vi "5_kb_plot_main.vi"() -> ()   [LabVIEW 2019]
uses:
  helper_vis/TypeDef_Velocity.ctl
  Shared VIs/TypeDef_TDMS_States.ctl
  <vilib>/myRIO/Common/Instrument Driver Framework/myRIO v1.0/Encoder/typedefs/Encoder Signal Mode.ctl
  Shared VIs/ModelSpecific/ETHMikeModel.ctl
  Shared VIs/ModelSpecific/ReadOnlyGlobalActions.ctl
  <vilib>/myRIO/Instrument Drivers/Onboard IO/AI/typedefs/AI Reference.ctl
  <vilib>/myRIO/Common/Instrument Driver Framework/Utilities/typedefs/myRIO Generic Hardware Reference.ctl
  <vilib>/myRIO/Common/Instrument Driver Framework/Utilities/typedefs/Hardware Version Enum.ctl
  <vilib>/myRIO/Common/Instrument Driver Framework/Utilities/typedefs/myRIO v1.0 Reference.ctl
  <vilib>/myRIO/Common/Instrument Driver Framework/Utilities/typedefs/Generic FPGA Reference.ctl
  <vilib>/myRIO/Common/Instrument Driver Framework/myRIO v1.0/AI/typedefs/AI Channels List.ctl
  <vilib>/myRIO/Common/Instrument Driver Framework/myRIO v1.0/AI/typedefs/AI Channels Enum.ctl
  <vilib>/myRIO/Common/Instrument Driver Framework/Utilities/typedefs/Analog Scaling Constants List.ctl
  <vilib>/myRIO/Common/Instrument Driver Framework/Utilities/typedefs/Analog Scaling Constants.ctl
  <vilib>/userDefined/High Color/nirio_resource_hc.ctl
  <vilib>/myRIO/Instrument Drivers/Onboard IO/AO/typedefs/AO Reference.ctl
  <vilib>/myRIO/Common/Instrument Driver Framework/myRIO v1.0/AO/typedefs/AO Channels List.ctl
  <vilib>/myRIO/Common/Instrument Driver Framework/myRIO v1.0/AO/typedefs/AO Channels Enum.ctl
  <vilib>/Platform/TimedLoop/XDataNode/timing_clust.ctl
  <vilib>/Platform/TimedLoop/XDataNode/nitl_modes.ctl
  <vilib>/Platform/TimedLoop/XDataNode/wakeup.ctl
  <vilib>/Analysis/3filter.llb/Filter Passband Type.ctl
  <vilib>/myRIO/Common/Instrument Driver Framework/myRIO v1.0/AI/vis/myRIO v1.1 Open AI.vi
  <vilib>/myRIO/Common/Instrument Driver Framework/myRIO v1.0/AO/vis/myRIO v1.1 Open AO.vi
  <vilib>/myRIO/Common/Instrument Driver Framework/Utilities/vis/Validate Channels.vi
  <vilib>/myRIO/Common/Instrument Driver Framework/myRIO v1.0/AI/vis/myRIO v1.0 Reserve AI.vi
  <vilib>/myRIO/Common/Instrument Driver Framework/myRIO v1.0/AO/vis/myRIO v1.0 Reserve AO.vi
  <vilib>/myRIO/Common/Instrument Driver Framework/myRIO v1.0/AI/vis/myRIO v1.0 Close AI.vi
  <vilib>/myRIO/Common/Instrument Driver Framework/myRIO v1.0/AO/vis/myRIO v1.0 Close AO.vi
  <vilib>/myRIO/Common/Instrument Driver Framework/myRIO v1.0/Encoder/vis/myRIO v1.0 Close Encoder.vi
  <vilib>/myRIO/Common/Instrument Driver Framework/myRIO v1.0/AI/vis/myRIO v1.0 Build MUX Configuration AI.vi
  <vilib>/myRIO/Common/Instrument Driver Framework/myRIO v1.0/Resource Manager/vis/myRIO v1.0 Reserve Channel List.vi
  <vilib>/myRIO/Common/Instrument Driver Framework/myRIO v1.0/AO/vis/myRIO v1.0 Build MUX Configuration AO.vi
  <vilib>/myRIO/Common/Instrument Driver Framework/myRIO v1.0/AI/vis/myRIO v1.0 Unreserve AI.vi
  <vilib>/myRIO/Common/Instrument Driver Framework/myRIO v1.0/AO/vis/myRIO v1.0 Unreserve AO.vi
  <vilib>/myRIO/Common/Instrument Driver Framework/myRIO v1.0/Encoder/vis/myRIO v1.0 Unreserve Encoder.vi
  <vilib>/myRIO/Common/Instrument Driver Framework/myRIO v1.0/Resource Manager/vis/myRIO v1.0 Reserve Channel.vi
  <vilib>/myRIO/Common/Instrument Driver Framework/myRIO v1.0/Resource Manager/vis/myRIO v1.0 Unreserve Channel.vi
  <vilib>/myRIO/Common/Instrument Driver Framework/myRIO v1.0/Resource Manager/vis/myRIO v1.0 Unreserve Channel List.vi
  <vilib>/myRIO/Common/Instrument Driver Framework/myRIO v1.0/Encoder/vis/myRIO v1.0 Build MUX Configuration Encoder.vi
  <vilib>/myRIO/Common/Instrument Driver Framework/myRIO v1.0/Resource Manager/vis/myRIO v1.0 Build Mutex Name.vi
  <vilib>/myRIO/Common/Instrument Driver Framework/myRIO v1.0/Resource Manager/vis/myRIO v1.0 Create Configuration List.vi
  <vilib>/Utility/VariantDataType/GetNumericInfo.vi
  <vilib>/Utility/error.llb/Error Cluster From Error Code.vi
  <vilib>/myRIO/Common/Instrument Driver Framework/myRIO v1.0/myRIO v1.1 Open.vi
  <vilib>/myRIO/Common/Instrument Driver Framework/myRIO v1.0/AO/vis/myRIO v1.0 Get Scaling Constants AO.vi
  <vilib>/myRIO/Common/Instrument Driver Framework/Utilities/vis/IO Manager.vi
  <vilib>/myRIO/Common/Instrument Driver Framework/Utilities/vis/Configuration Manager.vi
  <vilib>/myRIO/Common/Instrument Driver Framework/myRIO v1.0/myRIO v1.0 Close.vi
  <vilib>/myRIO/Common/Instrument Driver Framework/myRIO v1.0/AO/vis/myRIO v1.0 Write AO.vi
  <vilib>/myRIO/Common/Instrument Driver Framework/myRIO v1.0/AI/vis/myRIO v1.0 Get Scaling Constants AI.vi
  <vilib>/myRIO/Common/Instrument Driver Framework/myRIO v1.0/AI/vis/myRIO v1.0 Read AI.vi
  <vilib>/myRIO/Common/Instrument Driver Framework/myRIO v1.0/Encoder/vis/myRIO v1.0 Read Encoder.vi
  <vilib>/myRIO/Common/Instrument Driver Framework/myRIO v1.0/Encoder/vis/myRIO v1.0 Enable Encoder.vi
  <vilib>/myRIO/Common/Instrument Driver Framework/myRIO v1.0/Encoder/vis/myRIO v1.0 Shutdown Encoder.vi
  <vilib>/myRIO/Common/Instrument Driver Framework/myRIO v1.0/Resource Manager/vis/myRIO v1.0 Configure IO.vi
  <vilib>/myRIO/Instrument Drivers/Onboard IO/AO/vis/myRIO AO Open.xnode
  <vilib>/myRIO/Instrument Drivers/Onboard IO/AI/vis/myRIO AI Open.xnode
  <vilib>/platform/TimedLoop/XDataNode/XDataNode.xnode
  <vilib>/myRIO/Instrument Drivers/Onboard IO/Encoder/Encoder.lvlib
  <vilib>/myRIO/Instrument Drivers/Onboard IO/AO/AO.lvlib
  <vilib>/Platform/TimedLoop/XDataNode/XDNodeRunTimeDep.lvlib
  <vilib>/myRIO/Instrument Drivers/Onboard IO/AI/AI.lvlib
  <vilib>/Analysis/NI_AALBase.lvlib
  <vilib>/ptbypt/NI_PtbyPt.lvlib
panel:
  in  "Torque Constant [Nm/A]":dbl=137.0 format="%#_13g"
  in  "TDMS Storage File Input":string
  out "TDMS States":T1
  in  "stop":bool
  out "Time (s)":dbl
  in  "Save data?":bool
  out "Force unfiltered":dbl
  out "Force [N]":dbl
  out "Force chart [N]":dbl(graph)
  out "Iteration Duration":i64
  in  "Velocity Method":T2
  in  "start rendering":bool
  out "Current Setpoint [A]":dbl
  out "Velocity [deg/s]":dbl
  out "Velocity [deg/s] Chart":dbl(graph)
  out "Current [A]":dbl
  out "Current [A] Chart":dbl(graph)
  out "Position [deg]":dbl
  out "Position [deg] Chart":dbl(graph)
  in  "Wall Position (deg)":dbl
  in  "B":dbl
  in  "K":dbl
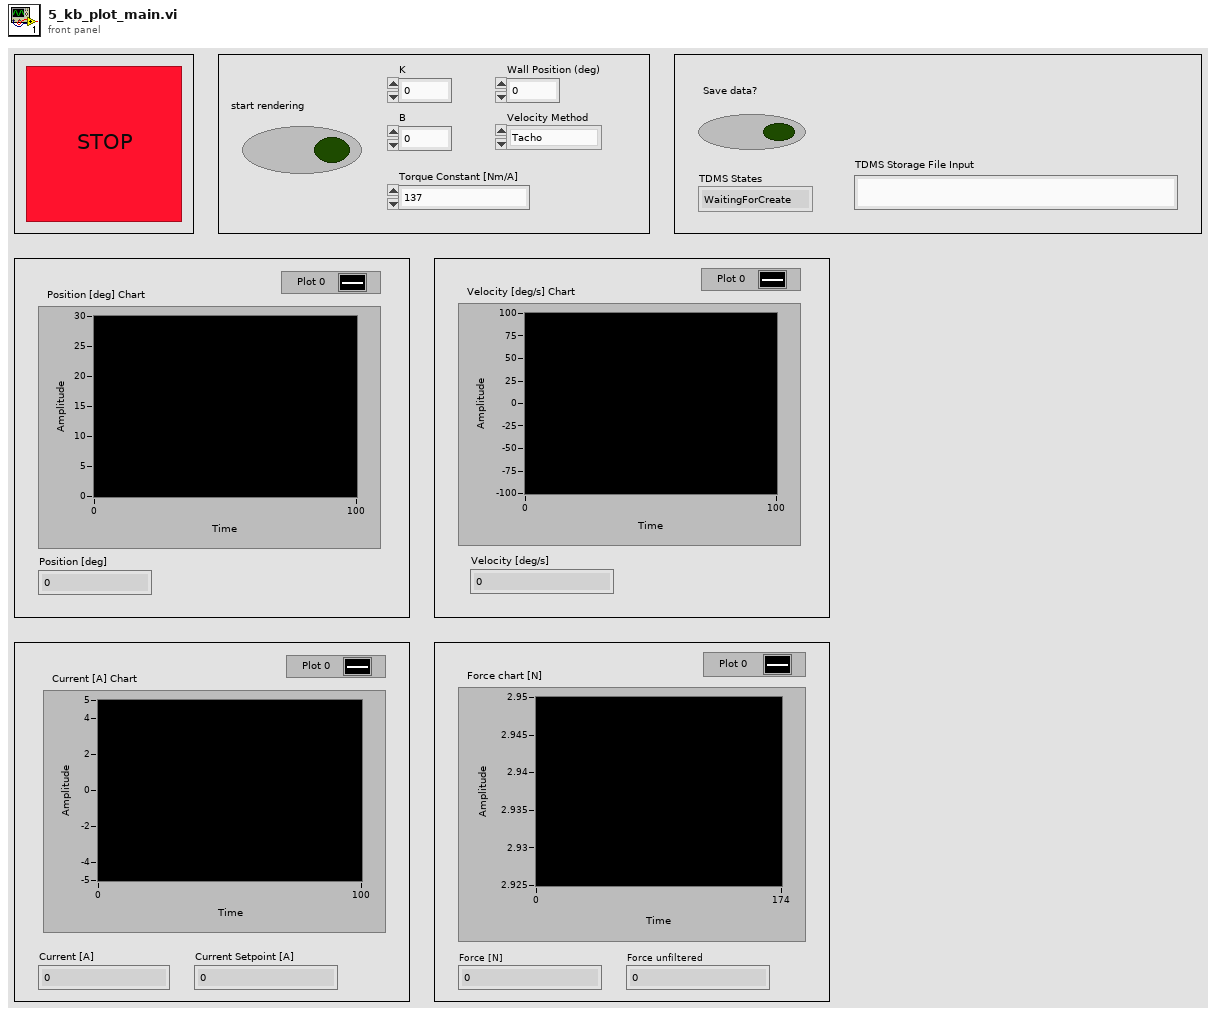
[diagram p1: front panel]
types:
  T1 = typedef "TypeDef_TDMS_States.ctl" = enum16{"WaitingForCreate", "Create", "Buffering", "Flushing", "Write", "Close"}
  T2 = typedef "TypeDef_Velocity.ctl" = enum16{"Tacho", "Encoder LP", "Encoder FOAW"}
  T3 = typedef "nirio_resource_hc.ctl" = tag
  T4 = typedef "Hardware Version Enum.ctl" = enum16{"Unknown", "myRIO-1900", "myRIO-1950", "roboRIO", "NI ELVIS RIO CM", "ELVIS III"}
  T5 = enum16{"open", "open or create", "create or replace", "create", "open (read-only)"}
  T6 = typedef "XDNodeRunTimeDep.lvlib/timing_clust.ctl" = cluster{"Expected End [f-1]":u64, "Actual End [f-1]":u64, "Finished Late? [f-1]":bool, "Expected End [i-1]":u64, "Actual End [i-1]":u64, "Finished Late? [i-1]":bool, "Expected Start [i]":u64, "Actual Start [i]":u64, "Expected Start [f]":u64, "Actual Start [f]":u64, "Source Name":string, "Structure Name":string, "Period":i64, "Deadline":i64, "Offset":i64, "Start":i64, "Priority":i32, "Timeout":i32, "Mode":T7, "Wakeup Reason":T8, "Error":errorcluster, "Source Type":string, "Secondary Source Type":string, "Global End Time":u64, "Global Start Time":u64, "Frame Duration":u64, "Iteration Duration":u64, "Assigned CPU":i32, "I/O Scan Engine Mode":u32}
  T7 = typedef "XDNodeRunTimeDep.lvlib/nitl_modes.ctl" = enum32{"No Change", "Process missed periods, maintain original phase", "Discard missed periods, maintain original phase", "Process missed periods, ignore original phase", "Discard missed periods, ignore original phase"}
  T8 = typedef "XDNodeRunTimeDep.lvlib/wakeup.ctl" = enum32{"Normal", "Aborted", "Asynchronous wakeup", "Timing source error", "Timed loop error", "Timeout"}
  T9 = typedef "NI_AALBase.lvlib/Filter Passband Type.ctl" = enum32{"Lowpass", "Highpass", "Bandpass", "Bandstop"}
  T10 = typedef "ReadOnlyGlobalActions.ctl" = enum16{"Initialize", "Read", "Write"}
  T11 = typedef "ETHMikeModel.ctl" = enum16{"ETH Mike #1", "ETH Mike #2", "ETH Mike #3", "ETH Mike #4", "ETH MIKE #5"}
  T12 = typedef "Encoder Signal Mode.ctl" = enum16{"Quadrature phase signal", "Step and direction signal"}
  T13 = typedef "AO.lvlib/AO Reference.ctl" = cluster{"myRIO Reference":T14, "AO Channel List":T17, "AO Scaling Constant List":T19}
  T14 = typedef "myRIO Generic Hardware Reference.ctl" = cluster{"myRIO Model":T4, "myRIO Hardware Reference":T15}
  T15 = typedef "myRIO v1.0 Reference.ctl" = cluster{"Generic FPGA Reference":T16, "Allow multiple opens":bool}
  T16 = typedef "Generic FPGA Reference.ctl" = refnum<k20>
  T17 = typedef "AO Channels List.ctl" = T18[]
  T18 = typedef "AO Channels Enum.ctl" = enum16{"Not Connected", "AudioOut/Left", "AudioOut/Right", "C/AO0", "C/AO1", "A/AO0", "A/AO1", "B/AO0", "B/AO1"}
  T19 = typedef "Analog Scaling Constants List.ctl" = T20[]
  T20 = typedef "Analog Scaling Constants.ctl" = cluster{"LSB Weight (Volts)":dbl, "Offset (Volts)":dbl, "Signed?":bool}
  T21 = typedef "AI.lvlib/AI Reference.ctl" = cluster{"myRIO Reference":T14, "AI Channels List":T22, "AI Scaling Constants List":T19}
  T22 = typedef "AI Channels List.ctl" = T23[]
  T23 = typedef "AI Channels Enum.ctl" = enum16{"Not Connected", "AudioIn/Left", "AudioIn/Right", "C/AI0", "C/AI1", "A/AI0", "A/AI1", "A/AI2", "A/AI3", "A/AI4", "A/AI5", "A/AI6", "A/AI7", "B/AI0", "B/AI1", "B/AI2", "B/AI3", "B/AI4", "B/AI5", "B/AI6", "B/AI7", "AI/AI0", "AI/AI1", "AI/AI2", "AI/AI3", "A/AI0 (DIFF)", "A/AI1 (DIFF)", "A/AI2 (DIFF)", "A/AI3 (DIFF)", "B/AI0 (DIFF)", "B/AI1 (DIFF)", "B/AI2 (DIFF)", "B/AI3 (DIFF)"}
  T24 = typedef "Encoder.lvlib/Encoder Reference.ctl" = cluster{"myRIO Reference":T14, "Encoder Channels Enum":T25}
  T25 = typedef "Encoder Channels Enum.ctl" = enum16{"Not Connected", "C/ENC0", "C/ENC1", "A/ENC", "A/ENC0", "A/ENC1", "A/ENC2", "A/ENC3", "A/ENC4", "A/ENC5", "A/ENC6", "A/ENC7", "A/ENC8", "A/ENC9", "B/ENC", "B/ENC0", "B/ENC1", "B/ENC2", "B/ENC3", "B/ENC4", "B/ENC5", "B/ENC6", "B/ENC7", "B/ENC8", "B/ENC9", "DIO/ENC0", "DIO/ENC1", "DIO/ENC2", "DIO/ENC3", "DIO/ENC4"}
  T26 = typedef "TypeDefTachometerParam.ctl" = cluster{"Offset [V]":dbl, "Gain [deg/sV]":dbl}
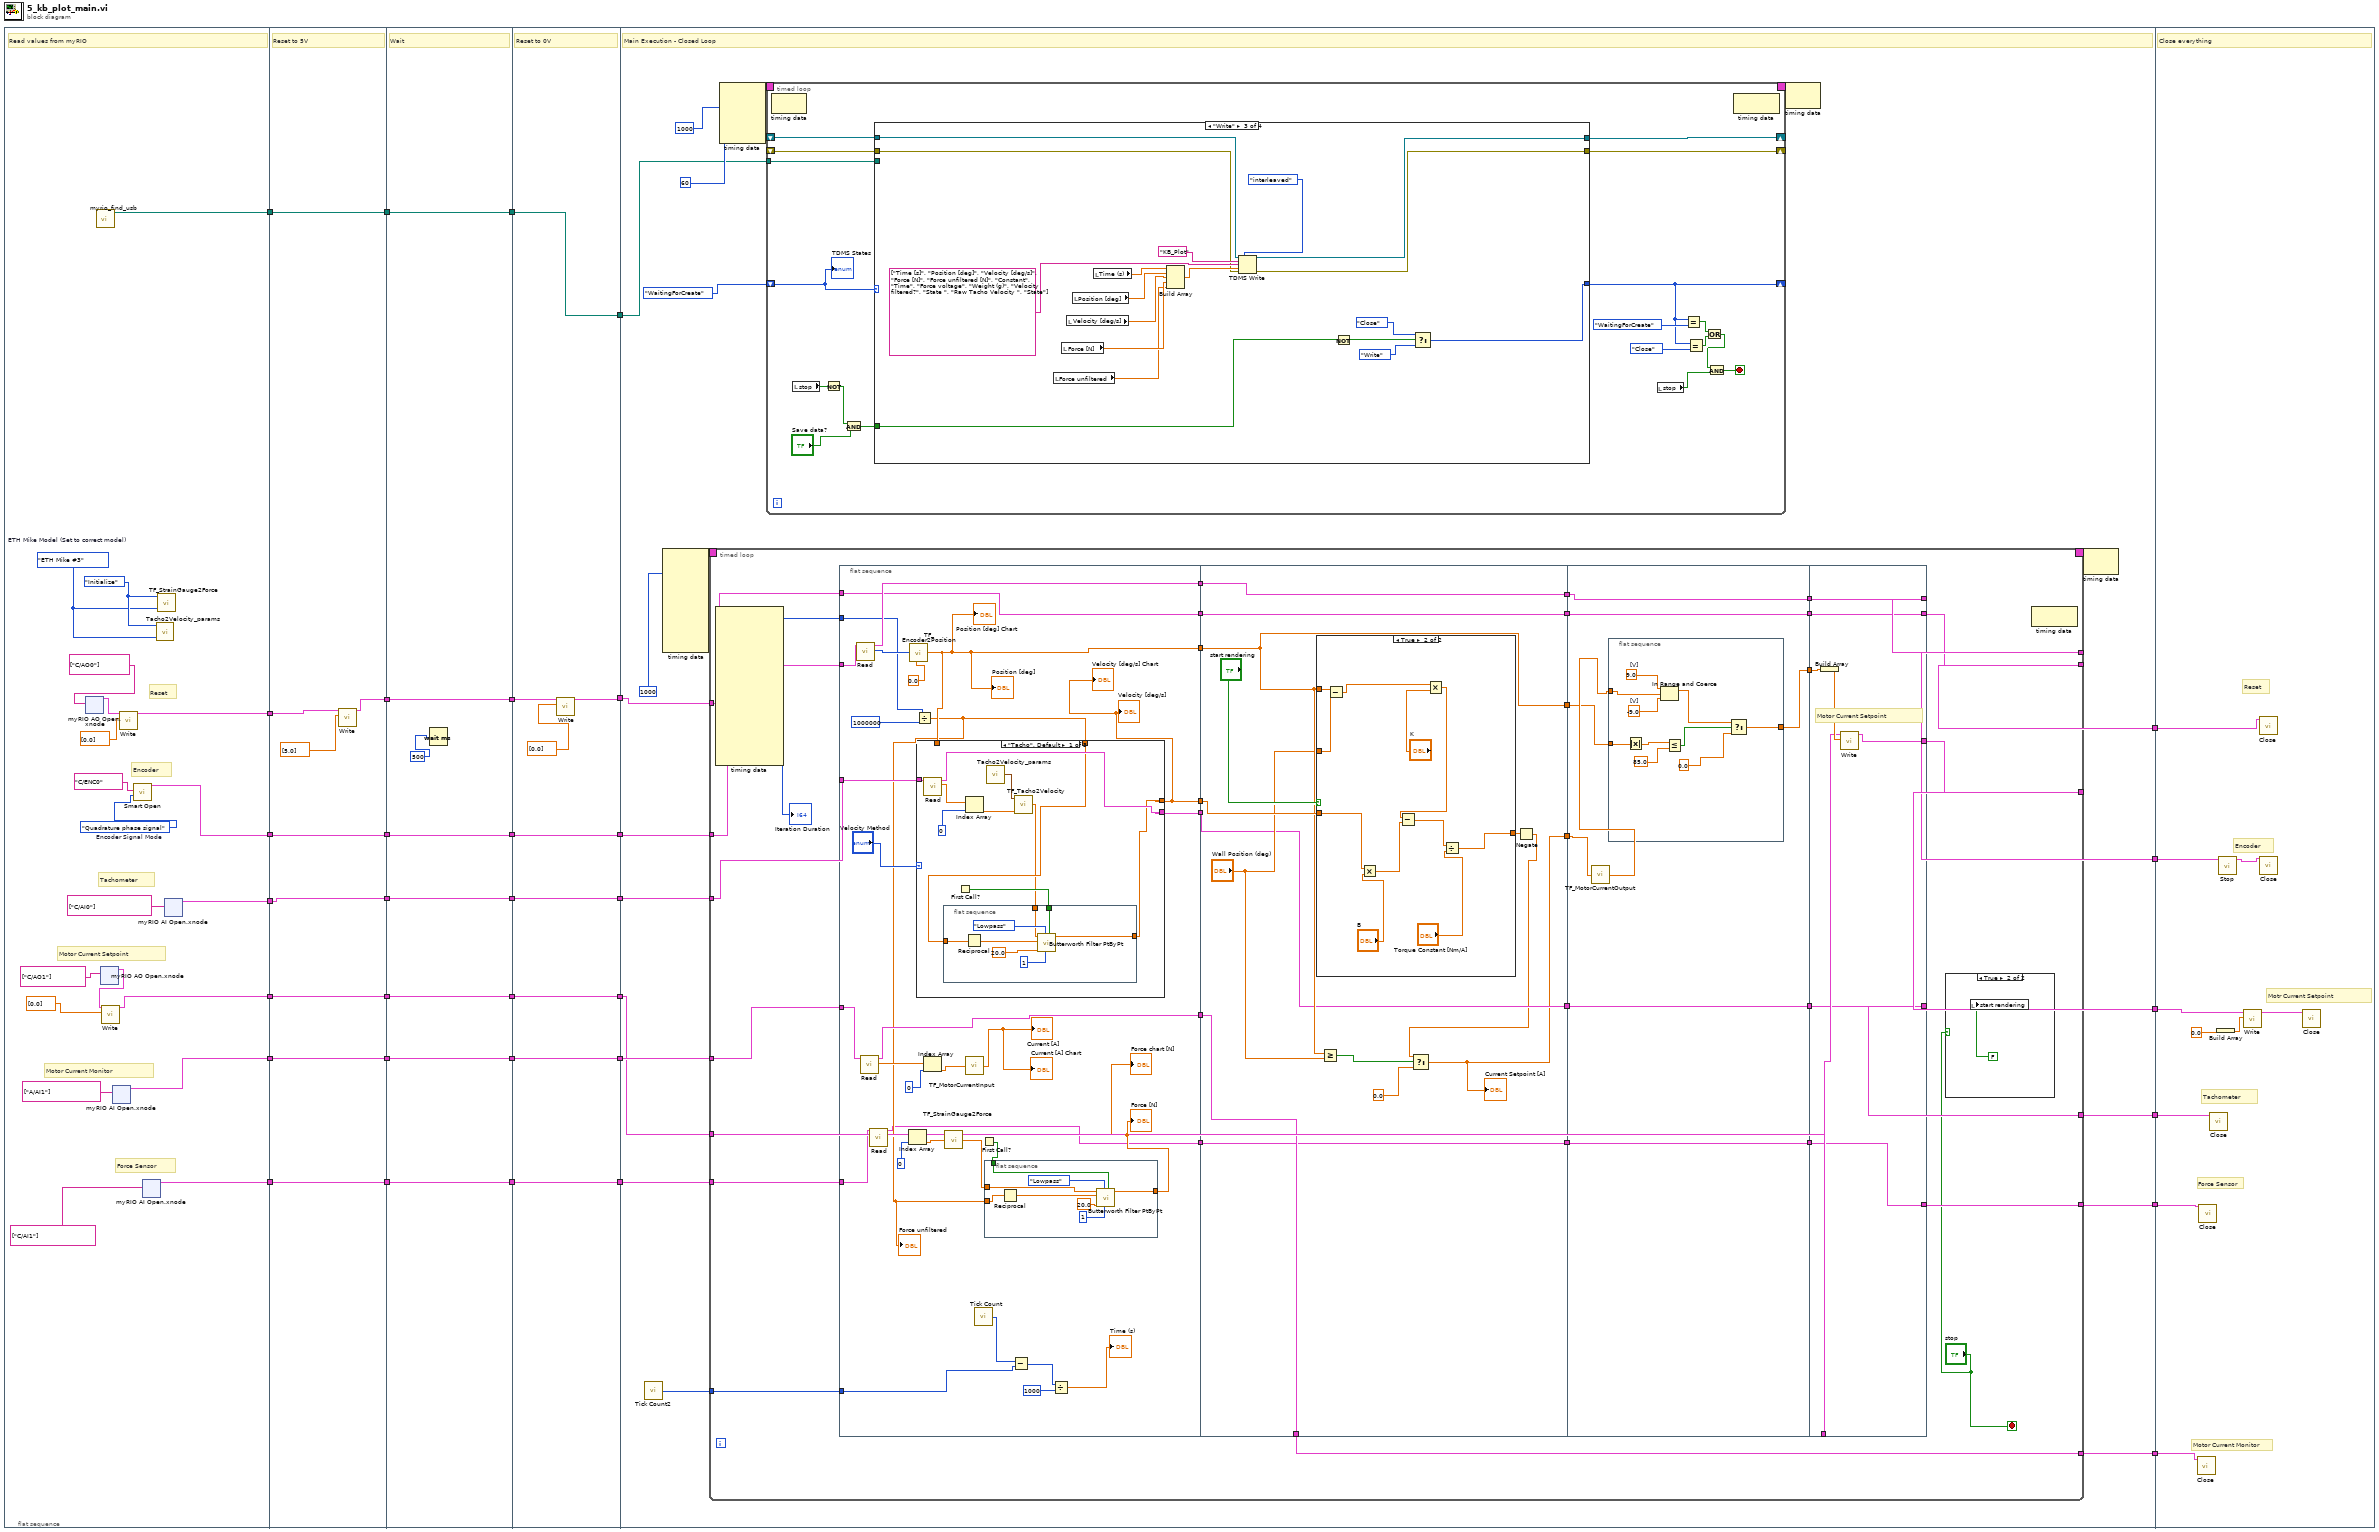
[diagram p0: block diagram]
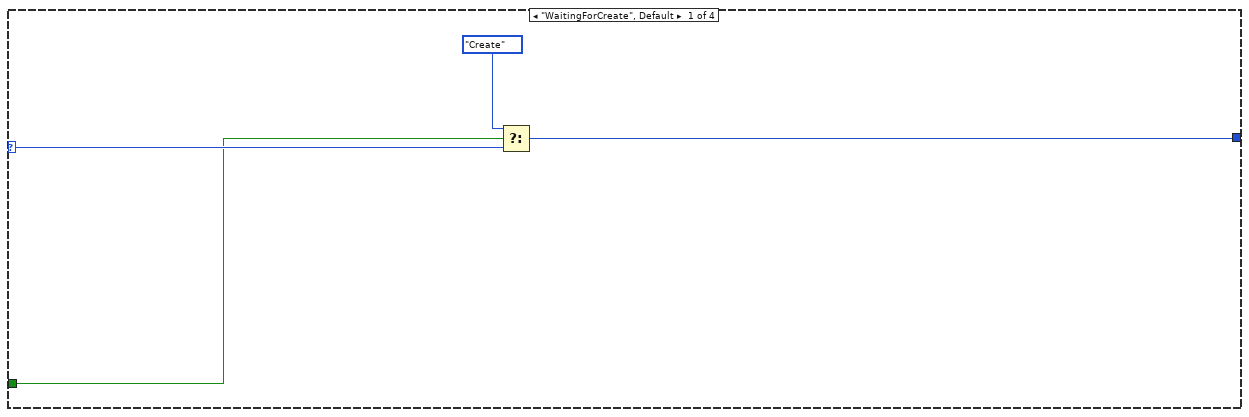
[diagram p2: hidden frame]
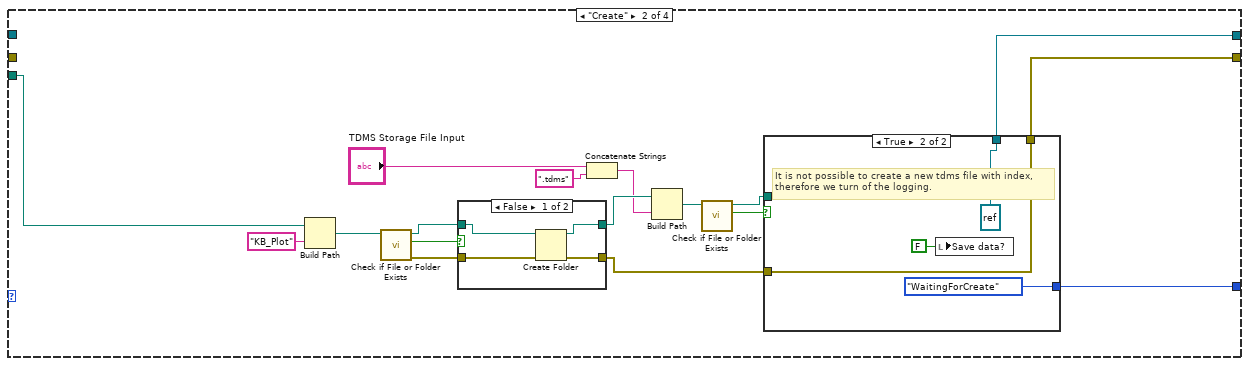
[diagram p3: hidden frame]
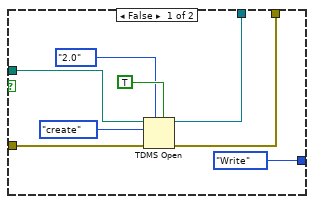
[diagram p4: hidden frame]
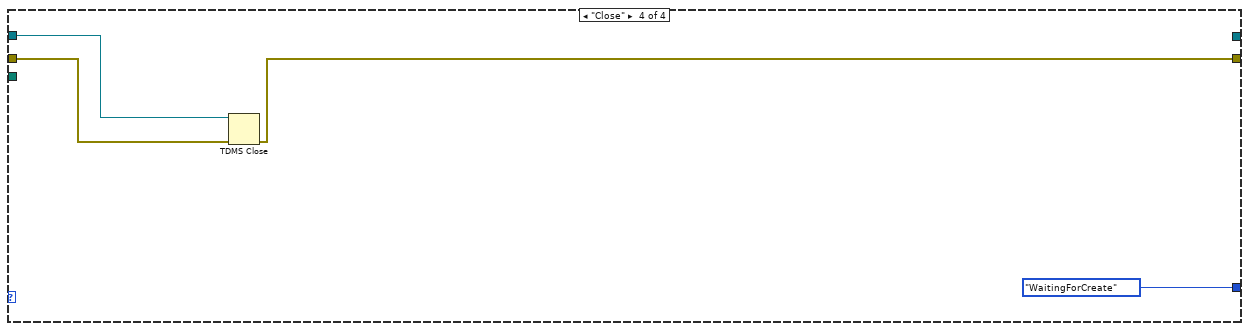
[diagram p6: hidden frame]
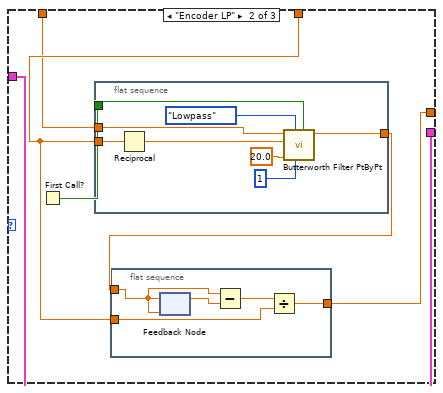
[diagram p8: hidden frame]
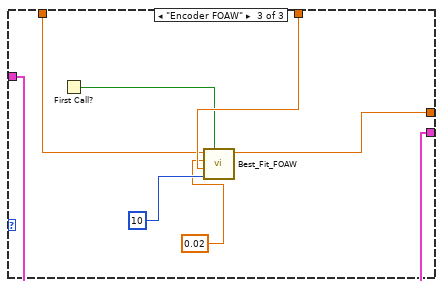
[diagram p9: hidden frame]
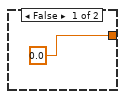
[diagram p10: hidden frame]
diagram:
  n1 = flat-sequence {
    tunnel: [w49] -> w34
    tunnel: [w48] -> w27
    tunnel: [w44] -> w26
    tunnel: [w42] -> w17
    tunnel: [w40] -> w16
    tunnel: [w38] -> w6
    tunnel: [w37] -> w2
    tunnel: w34 -> [w152]
    tunnel: [w151] -> w32
    tunnel: [w150] -> w28
    tunnel: w27 -> [w150]
    tunnel: w26 -> [w149]
    tunnel: [w149] -> w23
    tunnel: [w148] -> w18
    tunnel: w17 -> [w148]
    tunnel: w16 -> [w147]
    tunnel: [w147] -> w13
    tunnel: [w146] -> w7
    tunnel: w6 -> [w146]
    tunnel: [w145] -> w3
    tunnel: w2 -> [w145]
    tunnel: [w160] -> w33
    tunnel: w32 -> [w160]
    tunnel: [w159] -> w29
    tunnel: w28 -> [w159]
    tunnel: [w158] -> w24
    tunnel: w23 -> [w158]
    tunnel: [w157] -> w19
    tunnel: w18 -> [w157]
    tunnel: [w156] -> w14
    tunnel: w13 -> [w156]
    tunnel: [w155] -> w8
    tunnel: w7 -> [w155]
    tunnel: [w154] -> w4
    tunnel: w3 -> [w154]
    tunnel: w33 -> [w169]
    tunnel: [w168] -> w31
    tunnel: [w167] -> w30
    tunnel: w29 -> [w167]
    tunnel: [w166] -> w25
    tunnel: w24 -> [w166]
    tunnel: [w165] -> w20
    tunnel: w19 -> [w165]
    tunnel: [w164] -> w15
    tunnel: w14 -> [w164]
    tunnel: [w163] -> w9
    tunnel: w8 -> [w163]
    tunnel: [w162] -> w5
    tunnel: w4 -> [w162]
    tunnel: w31 -> [w183]
    tunnel: w30 -> [w189]
    tunnel: w25 -> [w185]
    tunnel: [w182] -> w22
    tunnel: [w184] -> w21
    tunnel: w20 -> [w188]
    tunnel: w15 -> [w187]
    tunnel: [w186] -> w12
    tunnel: [w181] -> w11
    tunnel: [w180] -> w10
    tunnel: w9 -> [w179]
    tunnel: w5 -> [w174]
    tunnel: [w173] -> w1
    tunnel: w22 -> [w463]
    tunnel: w21 -> [w462]
    tunnel: w12 -> [w461]
    tunnel: w11 -> [w460]
    tunnel: w10 -> [w459]
    tunnel: w1 -> [w458]
    frame #0 {
      w36 = ReadOnlyGlobalActions."Initialize" ("Action (Read)")
      w35 = ETHMikeModel."ETH Mike #3"  # ETH Mike Model (Set to correct model)
      w53 = Encoder_Signal_Mode."Quadrature phase signal"  # Encoder Signal Mode
      # "Force Sensor"
      # "Tachometer"
      # "Motor Current Monitor"
      # "Motor Current Setpoint"
      # "Reset"
      # "Encoder"
      # "Read values from myRIO"
      n2 = xnode "myRIO AO Open.xnode"("Channel Names"=tag[] ["C/AO0"]) -> ("AO Ref Out"=w51:T13)  [unwired: 2 in, 1 out]
      n3 = call "myrio_find_usb.vi"() -> ("Largest USB Partition Path"=w37:path)  [unwired: 9 in, 2 out]
      n4 = xnode "myRIO AO Open.xnode"("Channel Names"=tag[] ["C/AO1"]) -> ("AO Ref Out"=w46:T13)  [unwired: 2 in, 1 out]
      n5 = call <vilib>:"Write.vi"("Values"=dbl[] [0.0], "AO Ref In"=w46) -> ("AO Ref Out"=w44:T13)  [unwired: 7 in, 1 out]
      n6 = xnode "myRIO AI Open.xnode"("Channel Names"=tag[] ["A/AI1"]) -> ("AI Ref Out"=w42:T21)  [unwired: 2 in, 1 out]
      n7 = call <vilib>:"Write.vi"("Values"=dbl[] [0.0], "AO Ref In"=w51) -> ("AO Ref Out"=w49:T13)  [unwired: 7 in, 1 out]
      n8 = call <vilib>:"Smart Open.vi"("Encoder Signal Mode"=w53, "Channel Name"=tag "C/ENC0") -> ("Encoder Ref Out"=w48:T24)  [unwired: 8 in, 1 out]
      n9 = xnode "myRIO AI Open.xnode"("Channel Names"=tag[] ["C/AI1"]) -> ("AI Ref Out"=w38:T21)  [unwired: 2 in, 1 out]
      n10 = call "Tacho2Velocity_params.vi"("Action (Read)"=w36, "ETH Mike Model"=w35) -> ()  [unwired: 3 in, 1 out]
      n11 = call "TF_StrainGauge2Force.vi"("Action (Read)"=w36, "ETH Mike Model"=w35) -> ()  [unwired: 3 in, 1 out]
      n12 = xnode "myRIO AI Open.xnode"("Channel Names"=tag[] ["C/AI0"]) -> ("AI Ref Out"=w40:T21)  [unwired: 2 in, 1 out]
    }
    frame #1 {
      # "Reset to 5V"
      n13 = call <vilib>:"Write.vi"("Values"=dbl[] [5.0], "AO Ref In"=w152) -> ("AO Ref Out"=w151:T13)  [unwired: 7 in, 1 out]
    }
    frame #2 {
      # "Wait"
      n14 = Wait (ms)(milliseconds to wait=500) -> ()  [unwired: 1 out]
    }
    frame #3 {
      # "Reset to 0V"
      n15 = call <vilib>:"Write.vi"("Values"=dbl[] [0.0], "AO Ref In"=w169) -> ("AO Ref Out"=w168:T13)  [unwired: 7 in, 1 out]
    }
    frame #4 {
      # "Main Execution - Closed Loop"
      n16 = call "Tick Count2"() -> ("Tick Count(mSec)"=w172:u32)
      n17 = node-c288(1000) -> (w192:T6)  [unwired: 9 in]
      n18 = timed-loop {
        timing: w192 -> [_]
        timing-out: [_] -> w191
        tunnel: w189 -> [w305]
        tunnel: w188 -> [w312]
        tunnel: w187 -> [w311]
        tunnel: [w306] -> w186
        tunnel: w185 -> [w304]
        tunnel: [w300] -> w184
        tunnel: w183 -> [w299]
        tunnel: [w295] -> w182
        tunnel: [w291] -> w181
        tunnel: [w289] -> w180
        tunnel: w179 -> [w286]
        tunnel: [w284] -> w173
        tunnel: w172 -> [w280]
        stop <- "stop" stop-if-true
        n19 = node-c288() -> (w290:i64, →"Iteration Duration":i64)  [unwired: 1 in, 15 out]
        n20 = flat-sequence {
          tunnel: w305 -> [w345]
          tunnel: w312 -> [w342]
          tunnel: w311 -> [w337]
          tunnel: [w330] -> w310
          tunnel: [w329] -> w309
          tunnel: [w336] -> w302
          tunnel: w299 -> [w335]
          tunnel: [w335] -> w296
          tunnel: [w334] -> w294
          tunnel: w290 -> [w333]
          tunnel: [w328] -> w288
          tunnel: w286 -> [w327]
          tunnel: [w319] -> w281
          tunnel: w280 -> [w317]
          tunnel: w310 -> [w407]
          tunnel: w309 -> [w411]
          tunnel: [w399] -> w308
          tunnel: [w407] -> w307
          tunnel: [w410] -> w303
          tunnel: w302 -> [w410]
          tunnel: [w409] -> w297
          tunnel: w296 -> [w409]
          tunnel: w294 -> [w401]
          tunnel: [w401] -> w292
          tunnel: [w402] -> w289
          tunnel: w288 -> [w402]
          tunnel: [w398] -> w282
          tunnel: w281 -> [w398]
          tunnel: w308 -> [w431]
          tunnel: w307 -> [w426]
          tunnel: w303 -> [w430]
          tunnel: [w430] -> w301
          tunnel: [w429] -> w298
          tunnel: w297 -> [w429]
          tunnel: [w428] -> w293
          tunnel: w292 -> [w428]
          tunnel: [w425] -> w285
          tunnel: [w424] -> w283
          tunnel: w282 -> [w424]
          tunnel: [w448] -> w306
          tunnel: w304 -> [w447]
          tunnel: [w446] -> w300
          tunnel: w301 -> [w446]
          tunnel: w298 -> [w445]
          tunnel: [w445] -> w295
          tunnel: [w444] -> w291
          tunnel: w293 -> [w444]
          tunnel: w285 -> [w443]
          tunnel: [w442] -> w284
          tunnel: w283 -> [w442]
          frame #0 {
            n21 = call <vilib>:"Read.vi"("Encoder Ref In"=w345) -> ("Counter Value"=w344:i32, "Encoder Ref Out"=w336:T24)  [unwired: 6 in, 3 out]
            n22 = call <vilib>:"Read.vi"("AI Ref In"=w342) -> ("Values"=w341:dbl[], "AI Ref Out"=w328:T21)  [unwired: 8 in, 1 out]
            n23 = call <vilib>:"Read.vi"("AI Ref In"=w327) -> ("Values"=w326:dbl[], "AI Ref Out"=w319:T21)  [unwired: 8 in, 1 out]
            n24 = Index Array(array=w326, index=0) -> (element=w324:dbl)
            n25 = call "TF_Encoder2Position.vi"("Counter Value"=w344, "Offset"=0.0) -> ("Position [deg]"=w330:dbl)  [unwired: 3 in]
            "Position [deg] Chart" <- w330
            "Position [deg]" <- w330
            n26 = Divide(x=w333, y=1000000) -> (x/y=w320:dbl)
            "Force unfiltered" <- w320
            n27 = case shown="\"Tacho\", Default" "Velocity Method" {
              tunnel: w337 -> [w363 w377 w391]
              tunnel: [w360 w377 w391] -> w334
              tunnel: w320 -> [w359 w375 w396]
              tunnel: [w357 w374 w392] -> w329
              tunnel: w330 -> [_ w373 w394]
              frame "Tacho", Default {
                n28 = call <vilib>:"Read.vi"("AI Ref In"=w363) -> ("Values"=w361:dbl[], "AI Ref Out"=w360:T21)  [unwired: 8 in, 1 out]
                n29 = flat-sequence {
                  tunnel: w359 -> [w370]
                  tunnel: [w366] -> w357
                  tunnel: w358 -> [w365]
                  tunnel: w354 -> [w364]
                  frame #0 {
                    n30 = Reciprocal(x=w370) -> (1/x=w371:dbl)
                    n31 = call <vilib>:"Butterworth Filter PtByPt.vi"("initialize"=w365, "order"=1, "filter type"=Filter_Passband_Type."Lowpass", "low cutoff freq: fl"=20.0, "sampling freq: fs"=w371, "x"=w364) -> ("Filtered x"=w366:dbl)  [unwired: 3 in, 1 out]
                  }
                }
                n32 = First Call?() -> (First Call?: T/F=w358:bool)
                n33 = Index Array(array=w361, index=0) -> (element=w355:dbl)
                n34 = call "Tacho2Velocity_params.vi"() -> ("Cluster"=w356:T26)  [unwired: 5 in]
                n35 = call "TF_Tacho2Velocity.vi"("Tachometer Voltage [V]"=w355, "Tachometer param"=w356) -> ("Tachometer Velocity [deg/s]"=w354:dbl)  [unwired: 2 in]
              }
              frame "Encoder LP" {
                n36 = First Call?() -> (First Call?: T/F=w376:bool)
                n37 = flat-sequence {
                  tunnel: w373 -> [w390]
                  tunnel: w375 -> [w388]
                  tunnel: w376 -> [w385]
                  tunnel: [w383] -> w372
                  frame #0 {
                    n38 = Reciprocal(x=w388) -> (1/x=w389:dbl)
                    n39 = call <vilib>:"Butterworth Filter PtByPt.vi"("initialize"=w385, "order"=1, "filter type"=Filter_Passband_Type."Lowpass", "low cutoff freq: fl"=20.0, "sampling freq: fs"=w389, "x"=w390) -> ("Filtered x"=w383:dbl)  [unwired: 3 in, 1 out]
                  }
                }
                n40 = flat-sequence {
                  tunnel: w375 -> [w380]
                  tunnel: [w379] -> w374
                  tunnel: w372 -> [w378]
                  frame #0 {
                    n41 = feedback #1(w378) -> (w382:dbl)
                    n42 = feedback-in #1(w378) -> ()
                    n43 = Subtract(x=w378, y=w382) -> (x-y=w381:dbl)
                    n44 = Divide(x=w381, y=w380) -> (x/y=w379:dbl)
                  }
                }
              }
              frame "Encoder FOAW" {
                n45 = First Call?() -> (First Call?: T/F=w393:bool)
                n46 = call "Best_Fit_FOAW.vi"("y_k"=w394, "d"=0.02, "T"=w396, "n_max"=10, "Initialize"=w393) -> ("vel estimation"=w392:dbl)  [unwired: 4 in, 1 out]
              }
            }
            "Velocity [deg/s]" <- w329
            "Velocity [deg/s] Chart" <- w329
            n47 = Index Array(array=w341, index=0) -> (element=w339:dbl)
            n48 = call "TF_StrainGauge2Force.vi"("Strain Gauge Value [V]"=w324) -> ("Force [N]"=w323:dbl)  [unwired: 4 in]
            n49 = call "TF_MotorCurrentInput.vi"("Motor Current Monitor Value [V]"=w339) -> ("Current [A]"=→"Current [A] Chart" →"Current [A]":dbl)
            n50 = call "Tick Count"() -> ("Tick Count(mSec)"=w318:u32)
            n51 = First Call?() -> (First Call?: T/F=w322:bool)
            n52 = flat-sequence {
              tunnel: w323 -> [w353]
              tunnel: [w348] -> w321
              tunnel: w320 -> [w347]
              tunnel: w322 -> [w346]
              frame #0 {
                n53 = Reciprocal(x=w347) -> (1/x=w352:dbl)
                n54 = call <vilib>:"Butterworth Filter PtByPt.vi"("initialize"=w346, "order"=1, "filter type"=Filter_Passband_Type."Lowpass", "low cutoff freq: fl"=20.0, "sampling freq: fs"=w352, "x"=w353) -> ("Filtered x"=w348:dbl)  [unwired: 3 in, 1 out]
              }
            }
            n55 = Subtract(x=w318, y=w317) -> (x-y=w316:u32)
            n56 = Divide(x=w316, y=u32 1000) -> (x/y=→"Time (s)":dbl)
            "Force [N]" <- w321
            "Force chart [N]" <- w321
          }
          frame #1 {
            n57 = case shown="True" "start rendering" {
              tunnel: w411 -> [_ w420]
              tunnel: [0.0 w415] -> w403
              tunnel: w407 -> [_ w414]
              tunnel: "Wall Position (deg)" -> [_ w413]
              frame False {
              }
              frame True {
                n58 = Subtract(x=w414, y=w413) -> (x-y=w422:dbl)
                n59 = Multiply(x=w420, y="B") -> (x*y=w418:dbl)
                n60 = Multiply(x=w422, y="K") -> (x*y=w421:dbl)
                n61 = Subtract(x=w421, y=w418) -> (x-y=w416:dbl)
                n62 = Divide(x=w416, y="Torque Constant [Nm/A]") -> (x/y=w415:dbl)
              }
            }
            n63 = Greater Or Equal?(x=w407, y="Wall Position (deg)") -> (x >= y?=w406:bool)
            n64 = Negate(x=w403) -> (-x=w400:dbl)
            n65 = Select(t=w400, s=w406, f=0.0) -> (s? t:f=w399:dbl)
            "Current Setpoint [A]" <- w399
          }
          frame #2 {
            n66 = call "TF_MotorCurrentOutput.vi"("Motor Current Setpoint [A]"=w431) -> ("Motor Current Setpoint [V]"=w427:dbl)
            n67 = flat-sequence {
              tunnel: w426 -> [w437]
              tunnel: w427 -> [w433]
              tunnel: [w432] -> w425
              frame #0 {
                w441 = -9.0  # [V]
                w440 = 9.0  # [V]
                n68 = Absolute Value(x=w437) -> (abs(x)=w438:dbl)
                n69 = In Range and Coerce(upper limit=w440, x=w433, lower limit=w441) -> (coerced(x)=w439:dbl)  [unwired: 1 out]
                n70 = Less Or Equal?(x=w438, y=85.0) -> (x <= y?=w435:bool)
                n71 = Select(t=w439, s=w435, f=0.0) -> (s? t:f=w432:dbl)
              }
            }
          }
          frame #3 {
            # "Motor Current Setpoint"
            n72 = Build Array(w443) -> (w449:dbl[])
            n73 = call <vilib>:"Write.vi"("Values"=w449, "AO Ref In"=w447) -> ("AO Ref Out"=w448:T13)  [unwired: 7 in, 1 out]
          }
        }
        n74 = case shown="True" "stop" {
          frame False {
          }
          frame True {
            n75 = local write "start rendering"(FALSE ("start measurement")) -> ()
          }
        }
        n76 = node-c288() -> ()  [unwired: 1 in, 1 out]
      }
      n77 = node-c288(i64 1000 ("Period"), 60) -> (w178:T6)  [unwired: 3 in]
      n78 = timed-loop {
        timing: w178 -> [_]
        timing-out: [_] -> w177
        tunnel: w174 -> [w210]
        shift-right: [w209] -> _
        shift-left: _ -> [w208]
        shift-right: [w207] -> _
        shift-left: _ -> [w206]
        shift-right: [w196] -> _
        shift-left: TypeDef_TDMS_States."WaitingForCreate" ("TDMS States") -> [w201]
        stop <- w193 stop-if-true
        n79 = node-c288() -> ()  [unwired: 1 in, 1 out]
        n80 = local read "stop"() -> (w205:bool)
        n81 = Not(x=w205) -> (.not. x?=w203:bool)
        n82 = And(x=w203, y="Save data?") -> (x .and. y?=w202:bool)
        n83 = case shown="\"Write\"" w201 {
          selector: w201 -> [w214 _ _ _]
          tunnel: w202 -> [w213 _ w251 _]
          tunnel: w210 -> [_ w222 _ _]
          tunnel: [_ w217 w256 w269] -> w209
          tunnel: w208 -> [_ _ w259 w270]
          tunnel: [_ w216 w255 _] -> w207
          tunnel: w206 -> [_ _ w258 w271]
          tunnel: [w211 w219 w250 TypeDef_TDMS_States."WaitingForCreate" ("TDMS States")] -> w196
          frame "WaitingForCreate", Default {
            n84 = Select(t=TypeDef_TDMS_States."Create" ("TDMS States"), s=w213, f=w214) -> (s? t:f=w211:T1)
          }
          frame "Create" {
            n85 = Build Path(base path=w222, name or relative path="KB_Plot") -> (appended path=w224:path)
            n86 = call <vilib>:"Check if File or Folder Exists.vi"("path"=w224) -> ("error out"=w229:errorcluster, "file or folder exists?"=w231:bool, "dup path"=w230:path)  [unwired: 8 in]
            n87 = case shown="False" w231 {
              tunnel: w230 -> [w247 w248]
              tunnel: [w246 w249] -> w218
              tunnel: w229 -> [w245 w249]
              tunnel: [w244 w248] -> w228
              frame False {
                n88 = Create Folder(path (use dialog)=w247, error in=w245) -> (created path=w244:path, error out=w246:errorcluster)  [unwired: 1 in, 1 out]
              }
              frame True {
              }
            }
            n89 = Concatenate Strings("TDMS Storage File Input", ".tdms") -> (w225:string)
            n90 = Build Path(base path=w228, name or relative path=w225) -> (appended path=w221:path)
            n91 = call <vilib>:"Check if File or Folder Exists.vi"("path"=w221) -> ("file or folder exists?"=w220:bool, "dup path"=w215:path)  [unwired: 8 in, 1 out]
            n92 = case shown="True" w220 {
              tunnel: [TypeDef_TDMS_States."Write" ("TDMS States") TypeDef_TDMS_States."WaitingForCreate" ("TDMS States")] -> w219
              tunnel: w218 -> [w235 w240]
              tunnel: [w234 w240] -> w217
              tunnel: [w233 refnum<k34> refnum ("tdms file out")] -> w216
              tunnel: w215 -> [w232 _]
              frame False {
                n93 = TDMS Open(5:TRUE, 7:enum16{"1.0", "2.0"}."2.0" ("file format version (2.0)"), 8:w235, 10:T5."create" ("operation (0:open)"), 11:w232) -> (0:w234:errorcluster, 3:w233:refnum<k34>)  [unwired: 2 in]
              }
              frame True {
                # "It is not possible to create a new tdms file with index,\ntherefore we turn of the logging."
                n94 = local write "Save data?"(FALSE ("Save data?")) -> ()
              }
            }
          }
          frame "Write" {
            n95 = local read "Force unfiltered"() -> (w263:dbl)
            n96 = local read "Force [N]"() -> (w264:dbl)
            n97 = local read "Velocity [deg/s]"() -> (w265:dbl)
            n98 = local read "Position [deg]"() -> (w266:dbl)
            n99 = local read "Time (s)"() -> (w267:dbl)
            n100 = Build Array(w267, w266, w265, w264, w263) -> (w262:dbl[])
            n101 = TDMS Write(0:w258, 1:enum16{"decimated", "interleaved"}."interleaved" ("data layout (0:decimated)"), 5:"KB_Plot" ("group name in (Untitled)"), 7:string[] ["Time [s]", "Position [deg]", "Velocity [deg/s]", "Force [N]", "Force unfiltered [N]", "Constant", "Time", "Force voltage", "Weight (g)", "Velocity filtered?", "State ", "Raw Tacho Velocity ", "State"], 9:w262, 11:w259) -> (4:w255:refnum<k34>, 15:w256:errorcluster)  [unwired: 2 out]
            n102 = Not(x=w251) -> (.not. x?=w254:bool)
            n103 = Select(t=TypeDef_TDMS_States."Close" ("TDMS States"), s=w254, f=TypeDef_TDMS_States."Write" ("TDMS States")) -> (s? t:f=w250:T1)
          }
          frame "Close" {
            n104 = TDMS Close(8:w270, 11:w271) -> (0:w269:errorcluster)  [unwired: 1 out]
          }
        }
        n105 = local read "stop"() -> (w194:bool)
        n106 = Equal?(x=w196, y=TypeDef_TDMS_States."WaitingForCreate" ("TDMS States")) -> (x = y?=w198:bool)
        n107 = Equal?(x=w196, y=TypeDef_TDMS_States."Close" ("TDMS States")) -> (x = y?=w197:bool)
        n108 = Or(x=w198, y=w197) -> (x .or. y?=w195:bool)
        n109 = And(x=w195, y=w194) -> (x .and. y?=w193:bool)
        n110 = node-c288() -> ()  [unwired: 1 in, 1 out]
        "TDMS States" <- w201
      }
      n111 = node-c288(w177) -> ()  [unwired: 1 out]
      n112 = node-c288(w191) -> ()  [unwired: 1 out]
    }
    frame #5 {
      # "Force Sensor"
      # "Motor Current Monitor"
      # "Tachometer"
      # "Reset"
      # "Encoder"
      # "Motr Current Setpoint"
      # "Close everything"
      n113 = call <vilib>:"Close.vi"("AI Ref In"=w459) -> ()  [unwired: 10 in, 1 out]
      n114 = call <vilib>:"Close.vi"("AI Ref In"=w458) -> ()  [unwired: 10 in, 1 out]
      n115 = call <vilib>:"Close.vi"("AI Ref In"=w460) -> ()  [unwired: 10 in, 1 out]
      n116 = Build Array(0.0) -> (w465:dbl[])
      n117 = call <vilib>:"Stop.vi"("Encoder Ref In"=w462) -> ("Encoder Ref Out"=w464:T24)  [unwired: 9 in, 1 out]
      n118 = call <vilib>:"Write.vi"("Values"=w465, "AO Ref In"=w461) -> ("AO Ref Out"=w467:T13)  [unwired: 7 in, 1 out]
      n119 = call <vilib>:"Close.vi"("AO Ref In"=w463) -> ()  [unwired: 10 in, 1 out]
      n120 = call <vilib>:"Close.vi"("Encoder Ref In"=w464) -> ()  [unwired: 10 in, 1 out]
      n121 = call <vilib>:"Close.vi"("AO Ref In"=w467) -> ()  [unwired: 10 in, 1 out]
    }
  }
